vi "Read Helper Stop Notifier.vi"(8 "error in (no error)":errorcluster, 11 "Helper Loop In":refnum<class "Helper Loop.lvclass">) -> (0 "error out":errorcluster, 2 "Helper Stopped Notifier":refnum<notifier>, 3 "Helper Loop Out":refnum<class "Helper Loop.lvclass">)   [LabVIEW 2020, in "Helper Loop.lvclass"]
doc: "Framework method for getting the notifier used to stop the helper loop and provide handshake that the loop has stopped."
uses:
  Helper Loop.lvclass
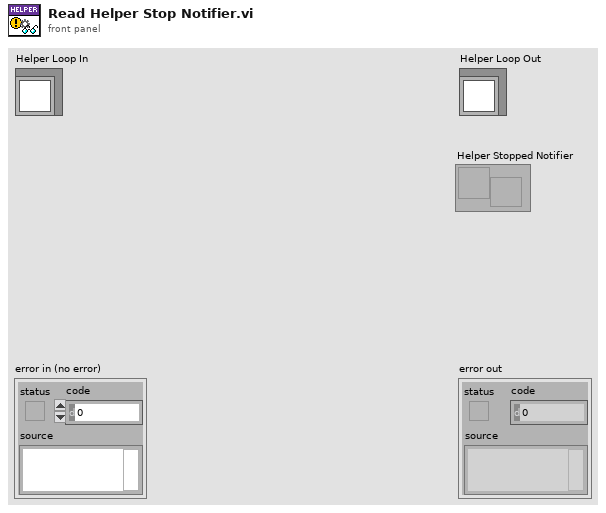
[diagram p1: front panel]
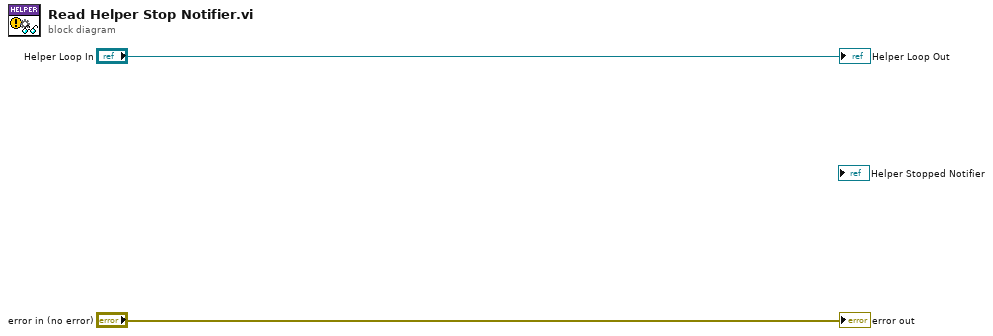
[diagram p0: block diagram]
diagram:
  "error out" <- "error in (no error)"
  "Helper Loop Out" <- "Helper Loop In"
